vi "DeviceInFIFO Write.vi"(8 "error in (no error)":errorcluster, 10 "DeviceInFIFO":refnum<k33>, 11 "DCM-NIVS-RT in":refnum<class "DCM-NIVS-RT.lvclass">) -> (0 "error out":errorcluster, 3 "DCM-NIVS-RT out":refnum<class "DCM-NIVS-RT.lvclass">)   [LabVIEW 2016, in "DCM Engine.lvlib" / "DCM-NIVS-RT.lvclass"]
uses:
  DCM-NIVS-RT.lvclass
  DCM-NIVS-RT.lvclass/DCM-NIVS-RT.ctl
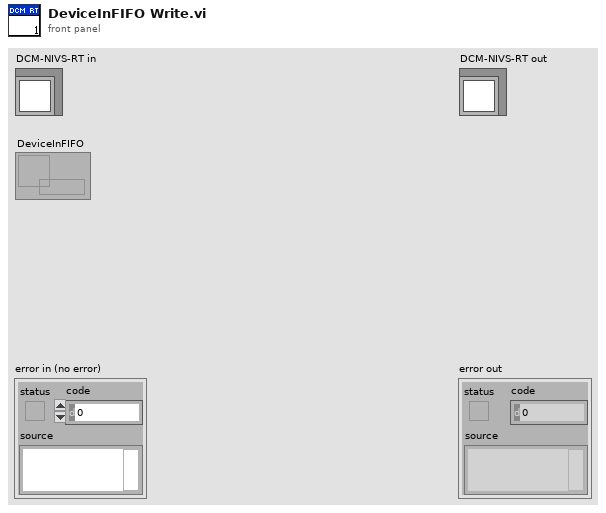
[diagram p1: front panel]
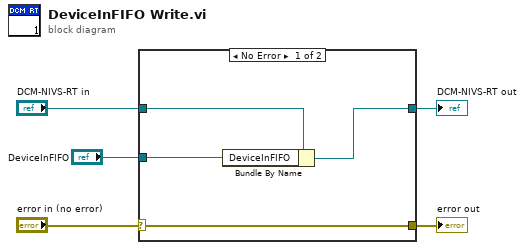
[diagram p0: block diagram]
diagram:
  n1 = case shown="No Error" "error in (no error)" {
    selector: "error in (no error)" -> [w9 w11]
    tunnel: [w9 w11] -> w4
    tunnel: [w7 w10] -> w2
    tunnel: "DCM-NIVS-RT in" -> [w8 w10]
    tunnel: "DeviceInFIFO" -> [w6 _]
    frame No Error {
      n2 = Bundle By Name(cluster=w8, "DeviceInFIFO"=w6) -> (w7:refnum<class "DCM-NIVS-RT.lvclass">)
    }
    frame Error {
    }
  }
  "error out" <- w4
  "DCM-NIVS-RT out" <- w2
